vi "表头数据.vi"(11 "选项":enum16{"初始化", "获取寄存器"}(ring)) -> (3 "表头输出":cluster{"DATA表头输出":string[], "ER表头输出":string[]})   [LabVIEW 2017]
uses:
  <vilib>/Utility/file.llb/Read Delimited Spreadsheet (string).vi
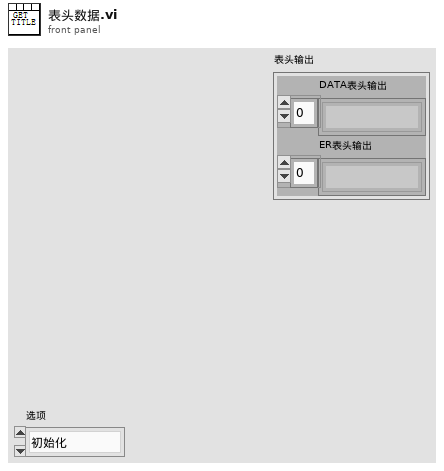
[diagram p1: front panel]
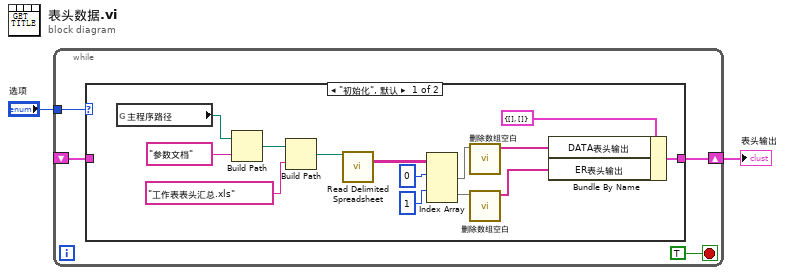
[diagram p0: block diagram]
diagram:
  n1 = while {
    tunnel: "选项" -> [w6]
    shift-right: [w5] -> w1
    shift-left: _ -> [w4]
    stop <- TRUE stop-if-true
    n2 = case shown="\"初始化\", 默认" w6 {
      tunnel: [w12 w21] -> w5
      tunnel: w4 -> [_ w21]
      frame "初始化", Default {
        n3 = global read "公共全局.vi" "主程序路径"() -> (w11:path)
        n4 = Build Path(base path=w11, name or relative path="参数文档" ("名称或相对路径")) -> (appended path=w9:path)
        n5 = Build Path(base path=w9, name or relative path="工作表表头汇总.xls" ("名称或相对路径")) -> (appended path=w7:path)
        n6 = call-poly <vilib>:"Read Delimited Spreadsheet.vi"("file path (dialog if empty)"=w7) -> ("all rows"=w20:string[][])  [unwired: 9 in, 5 out]
        n7 = Index Array(array=w20, index (row) #1=0 ("索引 (行)"), index (row) #2=1 ("索引 (行)")) -> (element #1=w16:string[], element #2=w17:string[])  [unwired: 2 in]
        n8 = call "删除数组空白.vi"("all rows输入"=w16) -> ("all rows输出"=w14:string[])  [unwired: 10 in]
        n9 = call "删除数组空白.vi"("all rows输入"=w17) -> ("all rows输出"=w13:string[])  [unwired: 10 in]
        n10 = Bundle By Name(cluster=cluster{"DATA表头输出":string[], "ER表头输出":string[]} {"DATA表头输出"=[], "ER表头输出"=[]}, "DATA表头输出"=w14, "ER表头输出"=w13) -> (w12:cluster{"DATA表头输出":string[], "ER表头输出":string[]})
      }
      frame "获取寄存器" {
      }
    }
  }
  "表头输出" <- w1
